vi "XY2 Macro.vi"(4 "X,Y Labels":string[](array[string])=["x label", "y label"], 6 "X,Y Log":i32[](array[numeric]), 8 "error in (no error)":errorcluster, 9 "Plot labels":string[](array[string])=["time", "V", "V^2", "V^3"], 10 "wavenames":string[](array[string])=["time.datatest.000005", "V.datatest.000005", "V^2.datatest.000005", "V^3.datatest.000005"], 11 "ITX Commands in":refnum<class "ITX Commands.lvclass">) -> (0 "error out":errorcluster, 2 "result string":string="Display/R 'time.datatest.000005'\nAppendToGraph 'V.datatest.000005'\nAppendToGraph 'V^2.datatest.000005'\nAppendToGraph 'V^3.datatest.000005'\nLabel bottom \"x label\"\nLabel left \"y label\"\nModifyGraph rgb('time.datatest.000005')=(65280,0,0)\nModifyGraph rgb('V.datatest.000005')=(41984,65280,0)\nModifyGraph rgb('V^2.datatest.000005')=(0,65280,45568)\nModifyGraph rgb('V^3.datatest.000005')=(2048,0,65280)\nLegend/C/N=text0/J \"\\\\s('time.datatest.000005') time\\r\\\\s('V.datatest.000005') V\\r\\\\s('V^2.datatest.000005') V^2\\r\\\\s('V^3.datatest.000005') V^3\"\nModifyGraph mirror=1\nModifyGraph width=216\nModifyGraph height={Aspect,0.6}\nModifyGraph Log(bottom)=0\nModifyGraph Log(left)=0\n", 3 "ITX Commands out":refnum<class "ITX Commands.lvclass">)   [LabVIEW 2019, in "ITX Commands.lvclass"]
uses:
  typedefs/Label--cluster.ctl
  typedefs/Log--cluster.ctl
  typedefs/log--enum.ctl
  ITX Commands.lvclass
panel:
  # "Legend/C/N=text0/J \"\\\\s('y_test.000011Plot9') Plot 9\\r\\\\s('y_test.000011Plot8') Plot 8\""
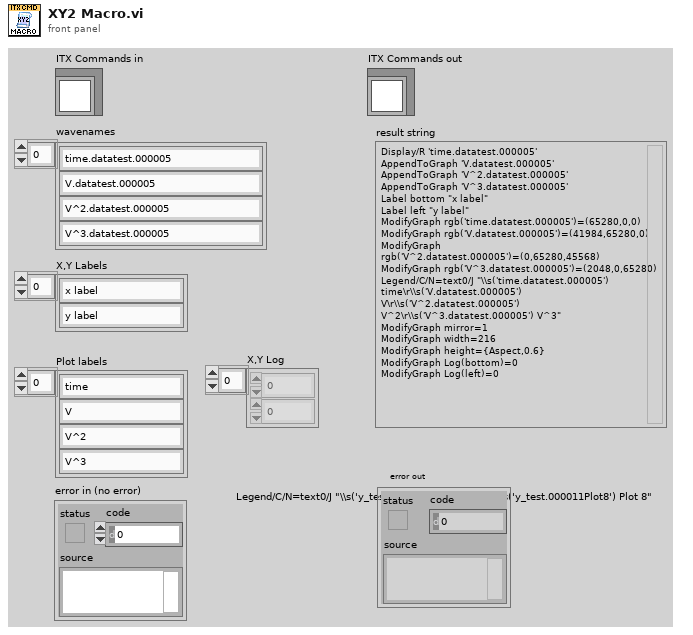
[diagram p1: front panel]
types:
  T1 = typedef "ITX Commands.lvclass/Log--cluster.ctl" = cluster{"bottom":T2, "left":T2}
  T2 = typedef "ITX Commands.lvclass/log--enum.ctl" = enum16{"normal axis", "log base 10", "log base 2"}
  T3 = typedef "ITX Commands.lvclass/Label--cluster.ctl" = cluster{"Bottom":string, "Top":string, "Left":string, "Right":string}
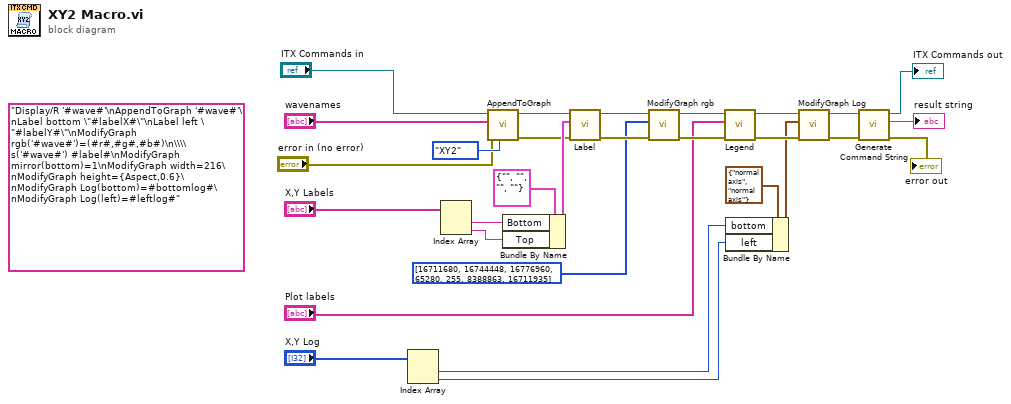
[diagram p0: block diagram]
diagram:
  (unwired) "Display/R '#wave#'\nAppendToGraph '#wave#'\nLabel bottom \"#labelX#\"\nLabel left \"#labelY#\"\nModifyGraph rgb('#wave#')=(#r#,#g#,#b#)\n\\\\s('#wave#') #label#\nModifyGraph mirror(bottom)=1\nModifyGraph width=216\nModifyGraph height={Aspect,0.6}\nModifyGraph Log(bottom)=#bottomlog#\nModifyGraph Log(left)=#leftlog#" ("input string")
  n1 = Index Array(array="X,Y Log") -> (element #1=w7:i32, element #2=w9:i32)  [unwired: 2 in]
  n2 = Index Array(array="X,Y Labels") -> (element #1=w24:string, element #2=w6:string)  [unwired: 2 in]
  n3 = call "AppendToGraph.vi"("Enum"=enum16{"XY", "XY2"}."XY2", "error in (no error)"="error in (no error)", "wavenames"="wavenames", "ITX Commands in"="ITX Commands in") -> ("error out"=w23:errorcluster, "ITX Commands out"=w25:refnum<class "ITX Commands.lvclass">)  [unwired: 6 in]
  n4 = Bundle By Name(cluster=T3 {"Bottom"="", "Top"="", "Left"="", "Right"=""} ("Label"), "Bottom"=w24, "Top"=w6) -> (w26:T3)
  n5 = call "Label.vi"("error in (no error)"=w23, "Label"=w26, "ITX Commands in"=w25) -> ("error out"=w21:errorcluster, "ITX Commands out"=w22:refnum<class "ITX Commands.lvclass">)  [unwired: 7 in]
  n6 = call "ModifyGraph rgb.vi"("error in (no error)"=w21, "Colorscale"=u32[] [16711680, 16744448, 16776960, 65280, 255, 8388863, 16711935], "ITX Commands in"=w22) -> ("error out"=w19:errorcluster, "ITX Commands out"=w18:refnum<class "ITX Commands.lvclass">)  [unwired: 7 in]
  n7 = call "Legend.vi"("error in (no error)"=w19, "Plot labels"="Plot labels", "ITX Commands in"=w18) -> ("error out"=w15:errorcluster, "ITX Commands out"=w14:refnum<class "ITX Commands.lvclass">)  [unwired: 7 in]
  n8 = Bundle By Name(cluster=T1 {"bottom"=enum."normal axis", "left"=enum."normal axis"} ("Log"), "bottom"=w7, "left"=w9) -> (w10:T1)
  n9 = call "ModifyGraph Log.vi"("error in (no error)"=w15, "Log"=w10, "ITX Commands in"=w14) -> ("error out"=w12:errorcluster, "ITX Commands out"=w13:refnum<class "ITX Commands.lvclass">)  [unwired: 7 in]
  n10 = call "Generate Command String.vi"("ITX Commands in"=w13, "error in (no error)"=w12) -> ("ITX Commands out"=→"ITX Commands out":refnum<class "ITX Commands.lvclass">, "ITX Commands"=→"result string":string, "error out"=→"error out":errorcluster)  [unwired: 6 in]
